vi "buildstring(sub).vi"(1 "Prefix":string, 2 "Command":dbl) -> (0 "Commandstring":string)   [LabVIEW 2015]
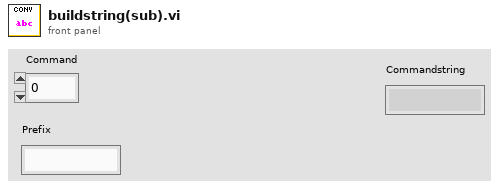
[diagram p1: front panel]
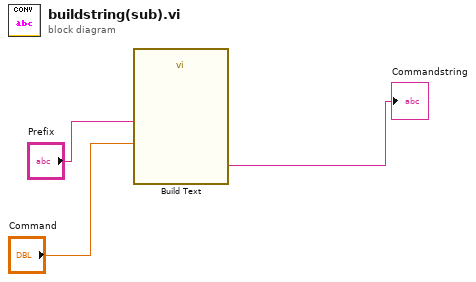
[diagram p0: block diagram]
diagram:
  n1 = call "Build Text"("Prefix"="Prefix", "Command"="Command") -> ("Result"=→"Commandstring":string)  [unwired: 12 in, 1 out]
